vi "FTW-File-AppendTimestampToFileName.vi"(1 "Format":T1=enum."YYYY-MM-DDT00-00-00 (simple locale)", 2 "Timestamp (unwired for current time)":timestamp format="%^<%Y-%m-%dT%H:%M:%S%3uZ>T", 7 "Path In":path) -> (8 "Path Out":path)   [LabVIEW 2015]
uses:
  Time/FTW-Time-DisplayFormat-Timestamp.ctl
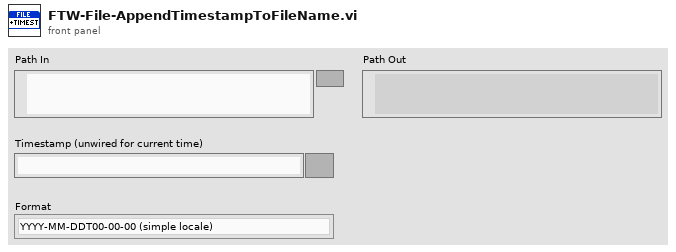
[diagram p1: front panel]
types:
  T1 = typedef "FTW-Time-DisplayFormat-Timestamp.ctl" = enum16{"YYYY-MM-DDT00:00:00.000Z (UTC)", "YYYY-MM-DDT00:00:00.000 (locale)", "YYYY-MM-DDT00:00:00.000+hh:mm (time zone)", "YYYY-MM-DDT00-00-00Z (simple UTC)", "YYYY-MM-DDT00-00-00 (simple locale)", "YYYY-MM-DD"}
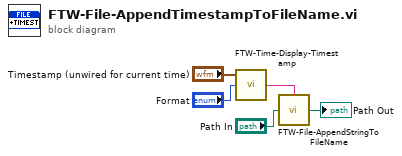
[diagram p0: block diagram]
diagram:
  n1 = call "FTW-Time-Display-Timestamp.vi"("Format"="Format", "Timestamp (unwired for current time)"="Timestamp (unwired for current time)") -> ("Formatted Timestamp"=w2:string)  [unwired: 2 in]
  n2 = call "FTW-File-AppendStringToFileName.vi"("String"=w2, "Path In"="Path In") -> ("Path Out"=→"Path Out":path)  [unwired: 13 in]
